vi "XML_Initilize.vi"(10 "User Input":string[](array[string])) -> (3 "DOM document out":refnum<k20>)   [LabVIEW 2009]
doc: "Sets up an XML file with HEADER and DATA_SET nodes as well as their child nodes. This VI is to be used to set up the XML_Data VI and should always be called before XML_Data.vi is called."
uses:
  <vilib>/xml/NI_XML.lvlib
panel:
  out "XML Output":string
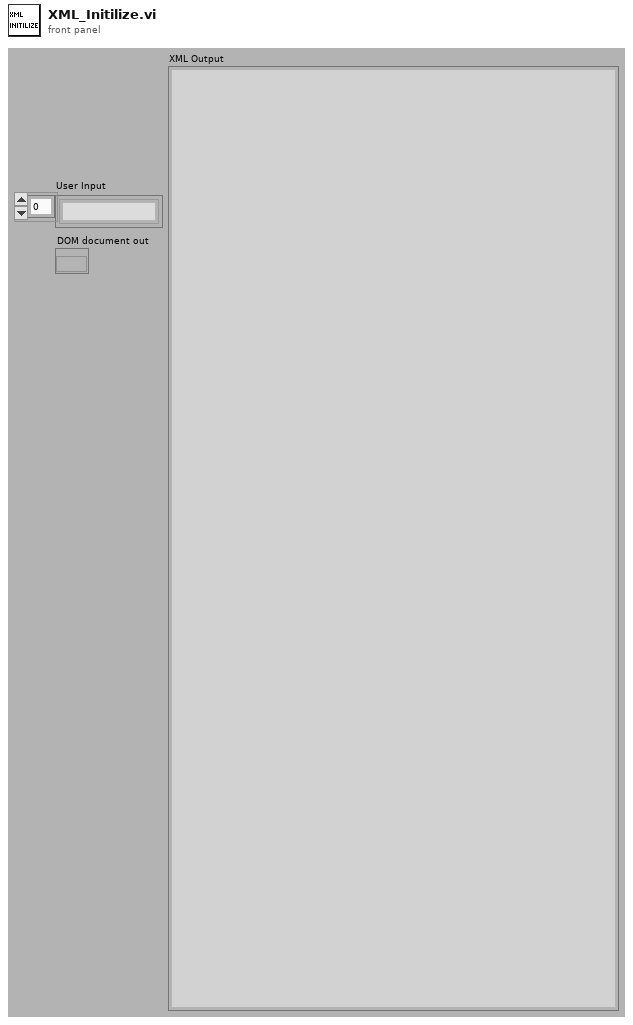
[diagram p1: front panel]
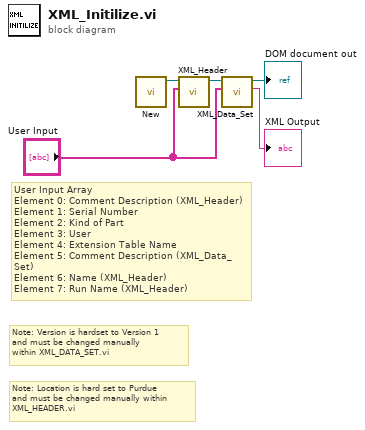
[diagram p0: block diagram]
diagram:
  # "User Input Array\nElement 0: Comment Description (XML_Header)\nElement 1: Serial Number\nElement 2: Kind of Part\nElement 3: User\nElement 4: Extension Table Name\nElement 5: Comment Description (XML_Data_Set)\nElement 6: Name (XML_Header)\nElement 7: Run Name (XML_Header)"
  # "Note: Location is hard set to Purdue\nand must be changed manually within \nXML_HEADER.vi"
  # "Note: Version is hardset to Version 1\nand must be changed manually \nwithin XML_DATA_SET.vi"
  n1 = call <vilib>:"New.vi"() -> ("DOM document out"=w4:refnum<k20>)  [unwired: 8 in, 1 out]
  n2 = call "XML_Header.vi"("User Input"="User Input", "DOM document in"=w4) -> ("OwnerDocument"=w3:refnum<k20>)  [unwired: 8 in, 1 out]
  n3 = call "XML_Data_Set.vi"("User Input"="User Input", "DOM document in"=w3) -> ("XML Output"=→"XML Output":string, "OwnerDocument"=→"DOM document out":refnum<k20>)  [unwired: 8 in]
